vi "sonar_foundwhale.vi"(1 "Current Position":i32, 2 "Sonar In":dbl) -> (0 "Found Whale":bool)   [LabVIEW 2014]
uses:
  <vilib>/Utility/file.llb/Read From Spreadsheet File (DBL).vi
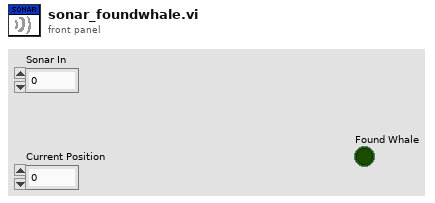
[diagram p1: front panel]
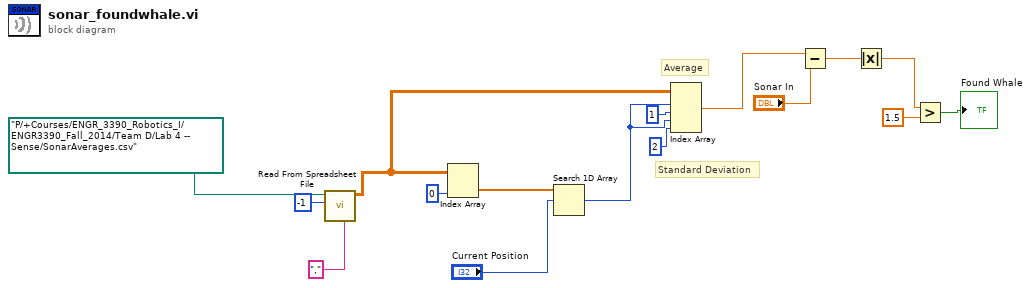
[diagram p0: block diagram]
diagram:
  # "Standard Deviation"
  # "Average"
  n1 = call-poly <vilib>:"Read From Spreadsheet File.vi"("delimiter (\\t)"="," ("delimiter (\\t)"), "number of rows (all:-1)"=-1, "file path (dialog if empty)"=path "P:/+Courses/ENGR_3390_Robotics_I/ENGR3390_Fall_2014/Team D/Lab 4 -- Sense/SonarAverages.csv") -> ("all rows"=w6:dbl[][])  [unwired: 4 in, 4 out]
  n2 = Index Array(array=w6, index (col)=0 ("disabled index (col)")) -> (element=w12:dbl[])  [unwired: 1 in]
  n3 = Search 1D Array(1D array=w12, element="Current Position") -> (index of element=w5:i32)  [unwired: 1 in]
  n4 = Index Array(array=w6, index (row) #1=w5, index (col) #1=1 ("index (col)"), index (row) #2=w5, index (col) #2=2 ("disabled index (col)")) -> (element #1=w9:dbl)  [unwired: 1 out]
  n5 = Subtract(x=w9, y="Sonar In") -> (x-y=w7:dbl)
  n6 = Absolute Value(x=w7) -> (abs(x)=w3:dbl)
  n7 = Greater?(x=w3, y=1.5) -> (0:→"Found Whale":bool)
